vi "__uintMultiply.vi"(8 "Base (decimal)":T1=10 items=["Binary"=2, "Octal"=8, "Decimal"=10, "Hexadecimal"=16, "Hexatrigesimal"=36, "ASCII"=64], 10 "UInt2 in":u8[](array[numeric])=[0], 11 "UInt1 in":u8[](array[numeric])=[0]) -> (0 "Timing multiplication":u32, 3 "UInt1 * Uint2":u8[](array[numeric]))   [LabVIEW 2011, in "UintClass.lvclass"]
uses:
  UintClass.lvclass
  enumBase.ctl
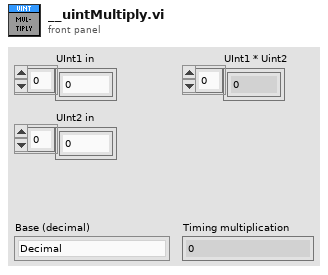
[diagram p1: front panel]
types:
  T1 = typedef "UintClass.lvclass/enumBase.ctl" = u16
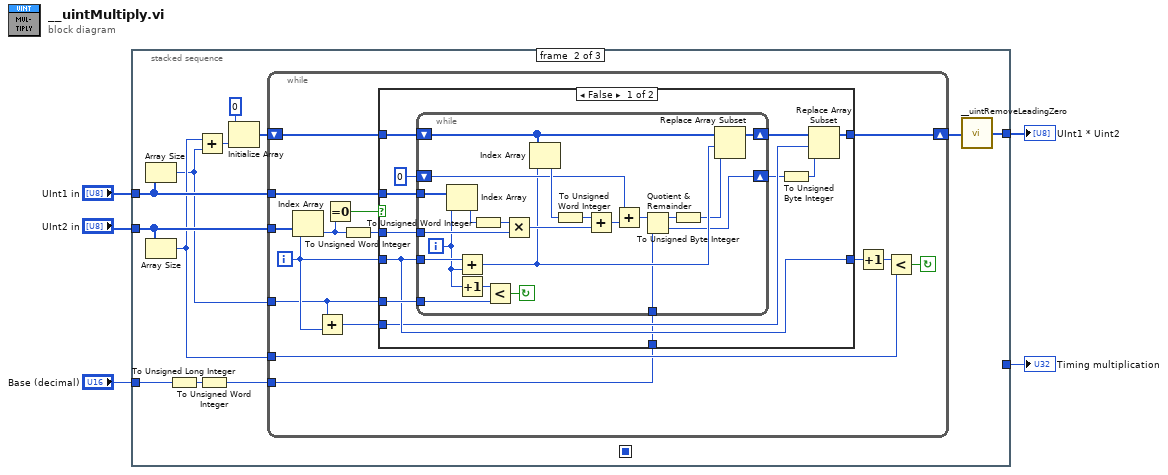
[diagram p0: block diagram]
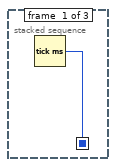
[diagram p2: hidden frame]
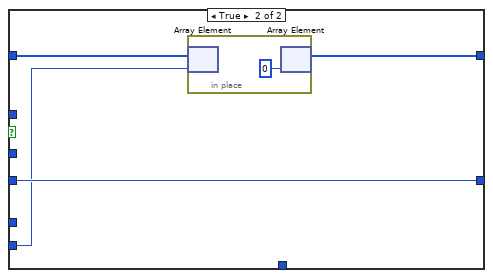
[diagram p3: hidden frame]
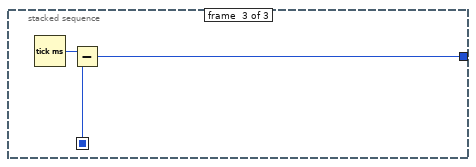
[diagram p4: hidden frame]
diagram:
  n1 = stacked-sequence {
    seq-local: [w6 _ _] -> [_ _ w73]
    tunnel: "UInt2 in" -> [_ w15 _]
    tunnel: "UInt1 in" -> [_ w14 _]
    tunnel: [_ w11 _] -> w3
    tunnel: "Base (decimal)" -> [_ w13 _]
    tunnel: [_ _ w74] -> w1
    frame #0 {
      n2 = Tick Count (ms)() -> (millisecond timer value=w6:u32)
    }
    frame #1 {
      n3 = Array Size(array=w14) -> (size(s)=w7:i32)
      n4 = Array Size(array=w15) -> (size(s)=w8:i32)
      n5 = To Unsigned Long Integer(number=w13) -> (unsigned 32bit integer=w10:u32)
      n6 = Add(x=w8, y=w7) -> (x+y=w18:i32)
      n7 = To Unsigned Word Integer(number=w10) -> (unsigned 16bit integer=w9:u16)
      n8 = Initialize Array(u8 0 ("element"), w18) -> (w17:u8[])
      n9 = while {
        tunnel: w15 -> [w26]
        tunnel: w14 -> [w25]
        tunnel: w7 -> [w23]
        shift-right: [w31] -> w12
        shift-left: w17 -> [w32]
        tunnel: w8 -> [w28]
        tunnel: w9 -> [w21]
        i -> [w24]
        stop <- w19 continue-if-true
        n10 = Index Array(array=w26, index=w24) -> (element=w27:u8)
        n11 = Add(x=w23, y=w24) -> (x+y=w22:i32)
        n12 = Equal To 0?(x=w27) -> (x = 0?=w33:bool)
        n13 = To Unsigned Word Integer(number=w27) -> (unsigned 16bit integer=w20:u16)
        n14 = case shown="False" w33 {
          tunnel: w32 -> [w42 w71]
          tunnel: w23 -> [w41 _]
          tunnel: w24 -> [w40 w69]
          tunnel: [w38 w70] -> w31
          tunnel: [w40 w69] -> w30
          tunnel: w25 -> [w44 _]
          tunnel: w20 -> [w43 _]
          tunnel: w22 -> [w37 w68]
          tunnel: w21 -> [w35 _]
          frame False {
            n15 = while {
              tunnel: w44 -> [w67]
              tunnel: w43 -> [w64]
              tunnel: w40 -> [w66]
              shift-right: [w55] -> w36
              shift-left: u16 0 -> [w60]
              tunnel: w41 -> [w51]
              shift-right: [w52] -> w39
              shift-left: w42 -> [w59]
              tunnel: w35 -> [w49]
              i -> [w54]
              stop <- w53 continue-if-true
              n16 = Index Array(array=w67, index=w54) -> (element=w65:u8)
              n17 = Add(x=w66, y=w54) -> (x+y=w58:i32)
              n18 = Increment(x=w54) -> (x+1=w50:i32)
              n19 = To Unsigned Word Integer(number=w65) -> (unsigned 16bit integer=w47:u16)
              n20 = Less?(x=w50, y=w51) -> (x < y?=w53:bool)
              n21 = Multiply(x=w47, y=w64) -> (x*y=w62:u16)
              n22 = Index Array(array=w59, index=w58) -> (element=w63:u8)
              n23 = To Unsigned Word Integer(number=w63) -> (unsigned 16bit integer=w48:u16)
              n24 = Add(x=w48, y=w62) -> (x+y=w61:u16)
              n25 = Add(x=w60, y=w61) -> (x+y=w57:u16)
              n26 = Quotient & Remainder(x=w57, y=w49) -> (x-y*floor(x/y)=w56:u16, floor(x/y)=w55:u16)
              n27 = To Unsigned Byte Integer(number=w56) -> (unsigned 8bit integer=w46:u8)
              n28 = Replace Array Subset(array=w59, new element=w46, index=w58) -> (w52:u8[])
            }
            n29 = To Unsigned Byte Integer(number=w36) -> (unsigned 8bit integer=w34:u8)
            n30 = Replace Array Subset(array=w39, new element=w34, index=w37) -> (w38:u8[])
          }
          frame True {
            n31 = in-place {
              n32 = in-place-array #1(w71, w68) -> ()  [unwired: 1 out]
              n33 = in-place-array #1(u8 0 ("element")) -> (w70:u8[])  [unwired: 1 out]
            }
          }
        }
        n34 = Increment(x=w30) -> (x+1=w29:i32)
        n35 = Less?(x=w29, y=w28) -> (x < y?=w19:bool)
      }
      n36 = call "__uintRemoveLeadingZero.vi"("Uint in"=w12) -> ("Uint out"=w11:u8[])
    }
    frame #2 {
      n37 = Tick Count (ms)() -> (millisecond timer value=w75:u32)
      n38 = Subtract(x=w75, y=w73) -> (x-y=w74:u32)
    }
  }
  "Timing multiplication" <- w1
  "UInt1 * Uint2" <- w3
